vi "Generate Cartesian Trajectory (Int).vi"(7 "intermediate points":i32, 8 "error in (no error)":errorcluster, 10 "end transform":T1, 11 "start transform":T1) -> (0 "error out":errorcluster, 3 "interpolated trajectory":dbl[][][](array[numeric]))   [LabVIEW 2017, in "NI_Kinematics.lvlib"]
doc: "Generates a smooth trajectory of end effector positions between two points in Cartesian space. Wire data to the <B>intermediate points</B> input to determine the polymorphic instance to use or manually select the instance.\n\n<B>.m file:</B> ctraj"
uses:
  <vilib>/robotics/Kinematics/NI_Kinematics.lvlib
  <vilib>/Analysis/Matrix/Datatypes/RealMatrix.ctl
  <vilib>/Analysis/Matrix/NI_Matrix.lvlib
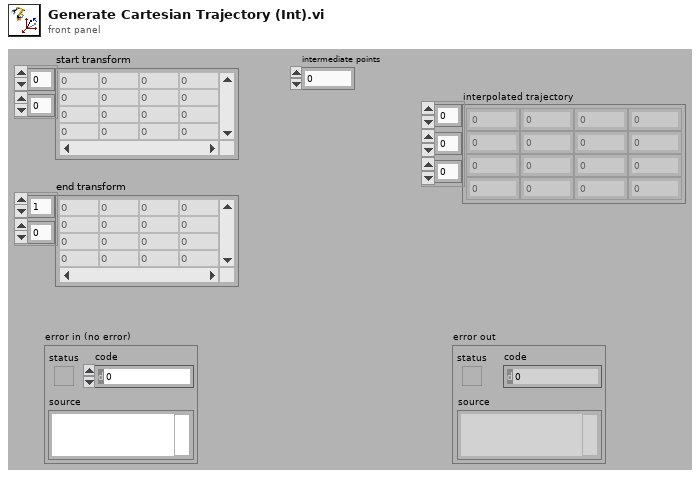
[diagram p1: front panel]
types:
  T1 = typedef "NI_Matrix.lvlib/RealMatrix.ctl" = dbl[][]
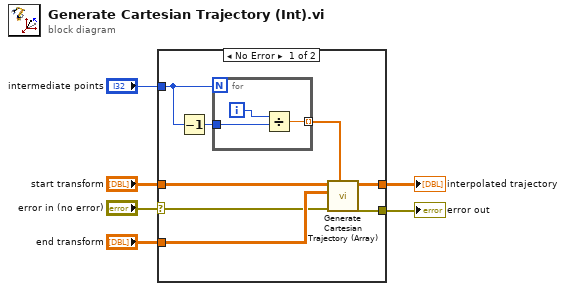
[diagram p0: block diagram]
diagram:
  n1 = case shown="No Error" "error in (no error)" {
    selector: "error in (no error)" -> [w7 w18]
    tunnel: "end transform" -> [w14 _]
    tunnel: "start transform" -> [w13 _]
    tunnel: [w12 _] -> w4
    tunnel: "intermediate points" -> [w11 _]
    tunnel: [w8 w18] -> w2
    frame No Error {
      n2 = Decrement(x=w11) -> (x-1=w10:i32)
      n3 = for {
        N: w11 -> [_]
        tunnel: w10 -> [w17]
        tunnel: [w15] -> w9 mode=indexing
        i -> [w16]
        n4 = Divide(x=w16, y=w17) -> (x/y=w15:dbl)
      }
      n5 = call <vilib>:"Generate Cartesian Trajectory (Array).vi"("intermediate points"=w9, "error in (no error)"=w7, "end transform"=w14, "start transform"=w13) -> ("error out"=w8:errorcluster, "interpolated trajectory"=w12:dbl[][][])  [unwired: 6 in]
    }
    frame Error {
    }
  }
  "interpolated trajectory" <- w4
  "error out" <- w2
